vi "Peek From Stack.vi"(8 "error in (no error)":errorcluster caption="错误输入（无错误）", 11 "Stack 输入":refnum<class "Stack.lvclass"> caption="DNL_LabVIEW Object in") -> (0 "error out":errorcluster caption="错误输出", 2 "Element":variant, 3 "Stack 输出":refnum<class "Stack.lvclass"> caption="DNL_LabVIEW Object out")   [LabVIEW 2011, in "Stack.lvclass"]
uses:
  Stack.lvclass
  Stack.lvclass/Stack.ctl
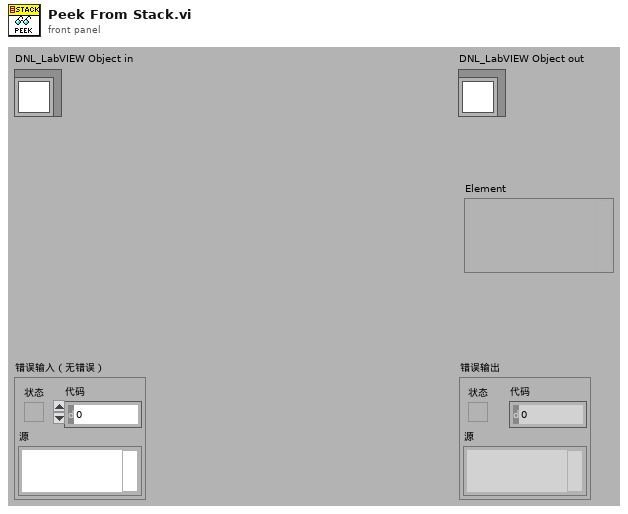
[diagram p1: front panel]
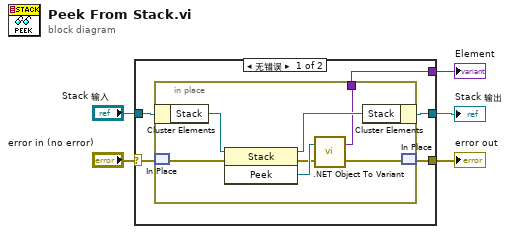
[diagram p0: block diagram]
diagram:
  n1 = case shown="无错误" "error in (no error)" {
    selector: "error in (no error)" -> [w10 w19]
    tunnel: [w6 w19] -> w4
    tunnel: [w8 w18] -> w2
    tunnel: "Stack 输入" -> [w9 w18]
    tunnel: [w7 _] -> w1
    frame No Error {
      n2 = in-place {
        in-place-border: [w12] -> w7
        n3 = in-place-cluster #1(w9) -> ("Stack"=w17:refnum<k24>)
        n4 = in-place-match #2(w10) -> (w15:errorcluster)
        n5 = invoke class="Stack" method="Peek"(reference=w17, error in=w15) -> (reference out=w16:refnum<k24>, error out=w13:errorcluster, "Peek"=w14:refnum<k24>)  [unwired: 1 in]
        n6 = call <vilib>:".NET Object To Variant.vi"("error in (no error)"=w13, ".NET object"=w14) -> ("error out"=w11:errorcluster, "variant"=w12:variant)
        n7 = in-place-cluster #1("Stack"=w16) -> (w8:refnum<class "Stack.lvclass">)
        n8 = in-place-match #2(w11) -> (w6:errorcluster)
      }
    }
    frame Error {
    }
  }
  "error out" <- w4
  "Stack 输出" <- w2
  "Element" <- w1
